vi "Frame_DATA_concept.vi"() -> ()   [LabVIEW 2024, in "PCANusb_DTU.lvlib"]
uses:
  PCANusb_DTU.lvlib
panel:
  out "unsigned byte array":u8[](array[numeric])
  out "Boolean array 3":bool[](array[boolean])
  out "(hi.lo)":u16
  out "*(type *) &x":u8[](array[numeric]) format="%.0x"
  out "appended array":bool[][](array[boolean])
  out "Boolean array 2":bool[](array[boolean])
  out "Boolean array":bool[][](array[boolean])
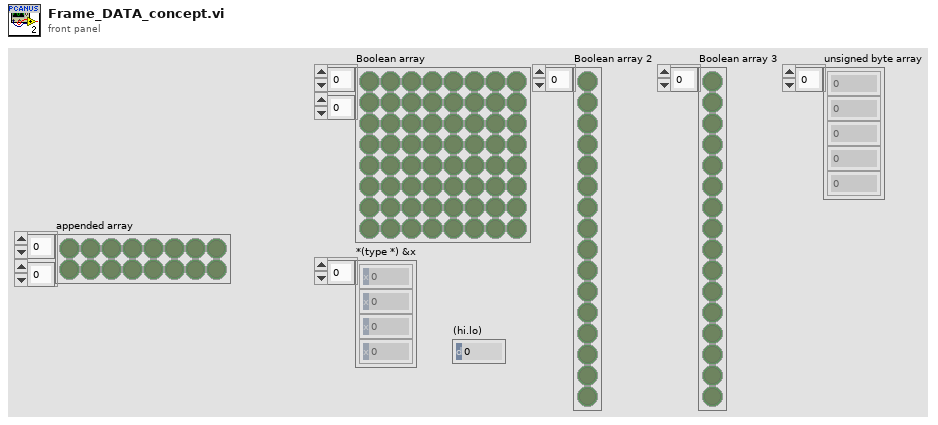
[diagram p1: front panel]
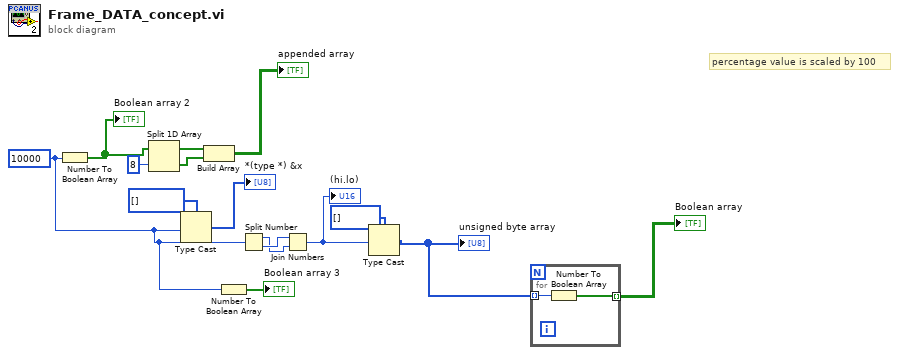
[diagram p0: block diagram]
diagram:
  w2 = u16 10000
  # "percentage value is scaled by 100"
  n1 = Number To Boolean Array(number=w2) -> (Boolean array=w14:bool[])
  "Boolean array 2" <- w14
  n2 = Split 1D Array(array=w14, index=8) -> (first subarray=w12:bool[], second subarray=w11:bool[])
  n3 = Type Cast(type=u8[] [], x=w2) -> (*(type *) &x=→"*(type *) &x":u8[])
  n4 = Build Array(w12, w11) -> (→"appended array":bool[][])
  n5 = Number To Boolean Array(number=w2) -> (Boolean array=→"Boolean array 3":bool[])
  n6 = Split Number(x=w2) -> (hi(x)=w6:u8, lo(x)=w7:u8)
  n7 = Join Numbers(hi=w7, lo=w6) -> ((hi.lo)=w1:u16)
  "(hi.lo)" <- w1
  n8 = Type Cast(type=u8[] [], x=w1) -> (*(type *) &x=w3:u8[])
  "unsigned byte array" <- w3
  n9 = for {
    tunnel: w3 -> [w17] mode=indexing
    tunnel: [w16] -> w15 mode=indexing
    n10 = Number To Boolean Array(number=w17) -> (Boolean array=w16:bool[])
  }
  "Boolean array" <- w15
